vi "RT1.vi"(8 "ErrorIn":errorcluster, 9 "Disconnect":bool) -> (0 "ErrorOut":errorcluster, 1 "Disconnected":bool)   [LabVIEW 2022 SP3]
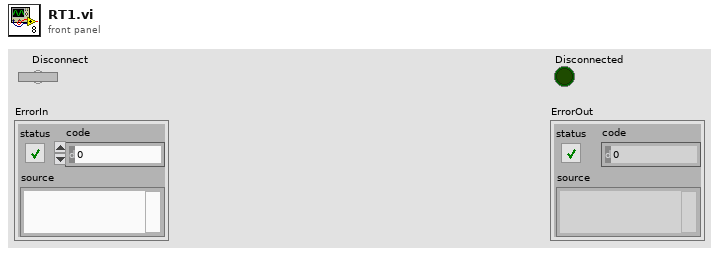
[diagram p1: front panel]
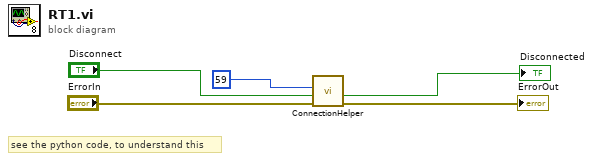
[diagram p0: block diagram]
diagram:
  # "see the python code, to understand this"
  n1 = call "ConnectionHelper.vi"("ErrorIn"="ErrorIn", "Disconnect"="Disconnect", "Setting"=u32 59) -> ("ErrorOut"=→"ErrorOut":errorcluster, "Disconnected"=→"Disconnected":bool)  [unwired: 6 in, 1 out]
